vi "Write Alarm.vi"(8 "error in (no error)":errorcluster, 10 "alarm":T1, 11 "NT Base in":refnum<class "NT Base.lvclass">) -> (0 "error out":errorcluster, 3 "NT Base out":refnum<class "NT Base.lvclass">)   [LabVIEW 2020, in "PV Access.lvlib" / "PV Data.lvlib" / "NT Base.lvclass"]
uses:
  NT Base.lvclass
  NT Base.lvclass/NT Base.ctl
  Alarm Severity.ctl
  PV Data.lvlib
  Alarm Status.ctl
  Alarm.ctl
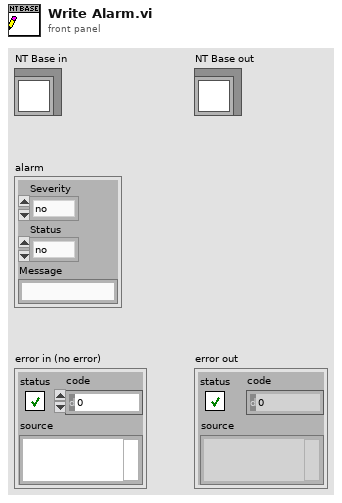
[diagram p1: front panel]
types:
  T1 = typedef "PV Access.lvlib/PV Data.lvlib/Alarm.ctl" = cluster{"Severity":T2, "Status":T3, "Message":string}
  T2 = typedef "PV Access.lvlib/PV Data.lvlib/Alarm Severity.ctl" = enum32{"no", "minor", "major", "record", "invalid", "undefined", ""}
  T3 = typedef "PV Access.lvlib/PV Data.lvlib/Alarm Status.ctl" = enum32{"no", "device", "driver", "record", "db", "conf", "undefined", "client"}
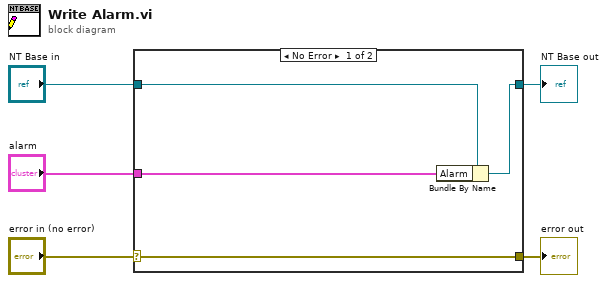
[diagram p0: block diagram]
diagram:
  n1 = case shown="No Error" "error in (no error)" {
    selector: "error in (no error)" -> [w9 w10]
    tunnel: [w9 w10] -> w4
    tunnel: [w7 w11] -> w2
    tunnel: "NT Base in" -> [w8 w11]
    tunnel: "alarm" -> [w6 _]
    frame No Error {
      n2 = Bundle By Name(cluster=w8, "Alarm"=w6) -> (w7:refnum<class "NT Base.lvclass">)
    }
    frame Error {
    }
  }
  "error out" <- w4
  "NT Base out" <- w2
